vi "enableRtAxis.vi"(8 "error":errorcluster, 9 "enabled":bool=TRUE, 10 "axis":i32, 11 "connection ID":refnum<k5>) -> (0 "error out":errorcluster, 2 "axis_out":i32, 3 "connection ID out":refnum<k5>)   [LabVIEW 2016, in "sen_api.lvlib"]
doc: "Sets the real-time output of the specific measurement axis."
uses:
  sen_api.lvlib
panel:
  out "jsonRespIn":string
  out "JSON-response":string="{\"jsonrpc\":\"2.0\",\"method\":\"\",\"params\":[5,1.245,true,\"name\"],\"id\":\"1\"}"
  out "JSON request":string
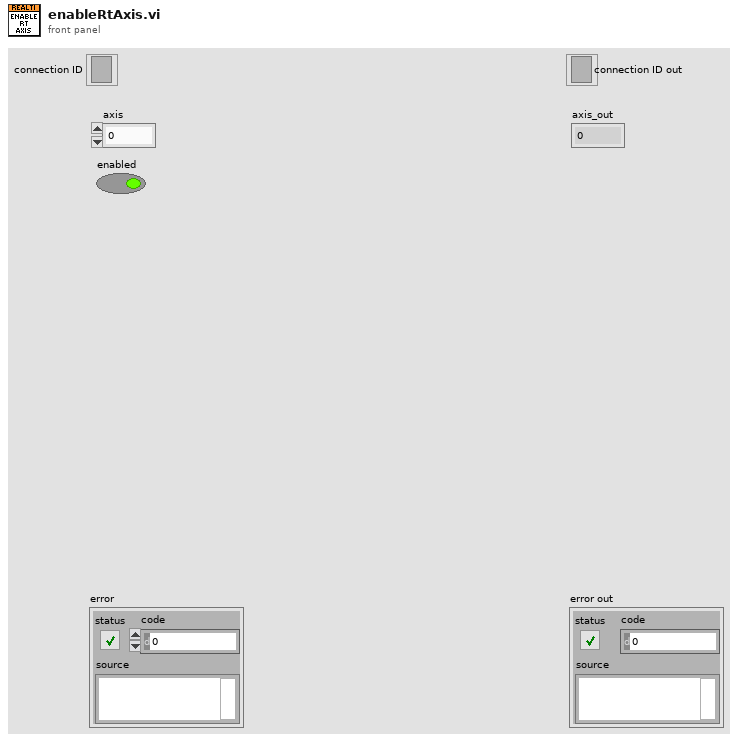
[diagram p1: front panel]
types:
  T1 = cluster{"jsonrpc":string, "method":string, "params":string[], "id":string, "api":i32, "pid":string}
  T2 = enum16{"Standard", "Buffered", "CRLF", "Immediate"}
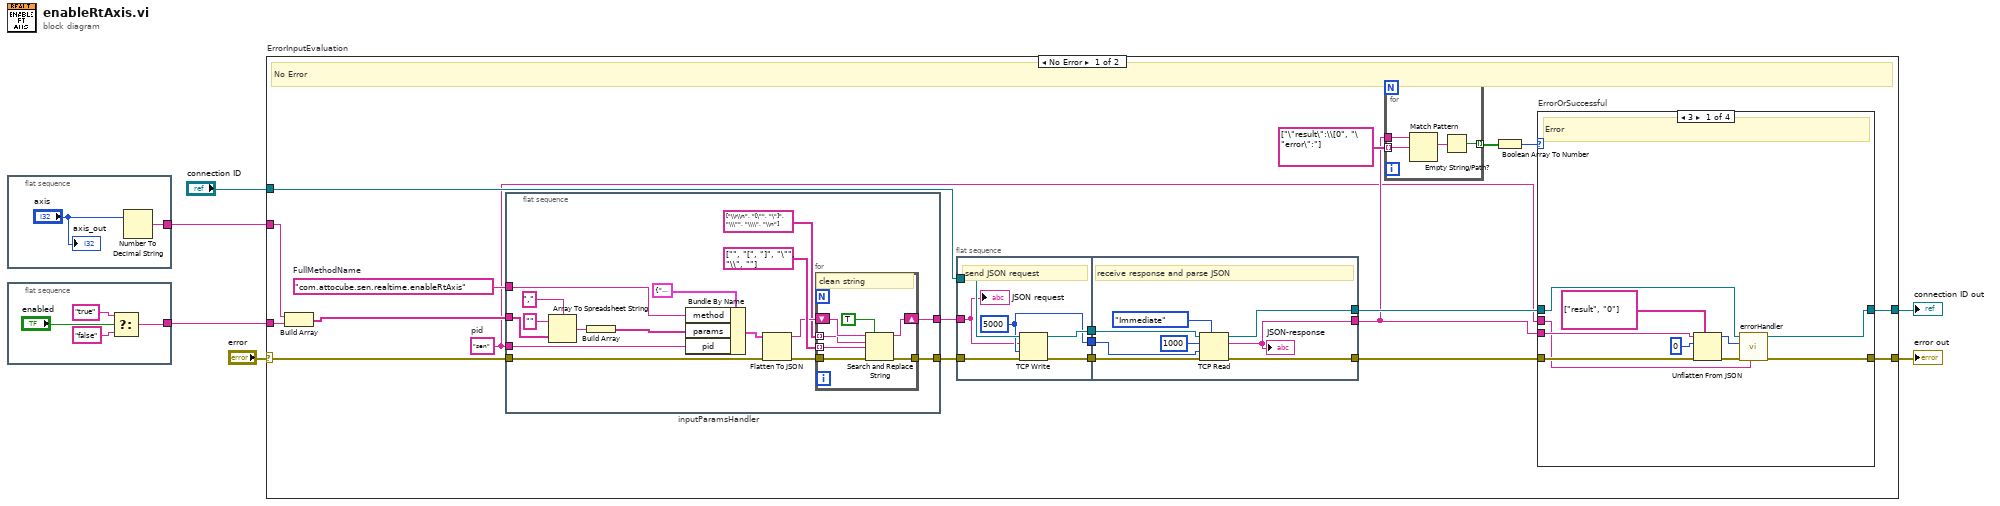
[diagram p0: block diagram]
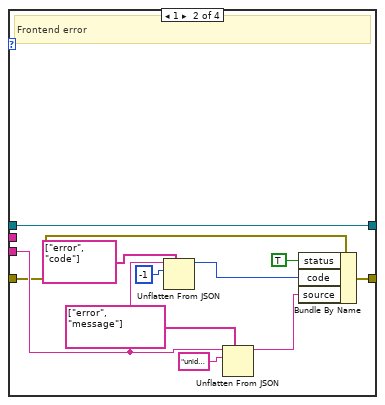
[diagram p2: hidden frame]
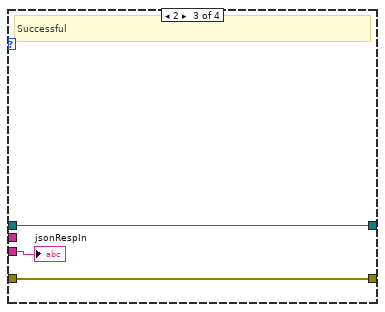
[diagram p3: hidden frame]
diagram:
  n1 = flat-sequence "in_axis" {
    tunnel: [w8] -> w2
    frame #0 {
      n2 = Number To Decimal String(number="axis") -> (decimal integer string=w8:string)  [unwired: 1 in]
      "axis_out" <- "axis"
    }
  }
  n3 = flat-sequence "in_bool" {
    tunnel: [w9] -> w1
    frame #0 {
      n4 = Select(t="true" ("Base"), s="enabled", f="false" ("Base")) -> (s? t:f=w9:string)
    }
  }
  n5 = case "ErrorInputEvaluation" shown="No Error" "error" {
    selector: "error" -> [w19 w100]
    tunnel: "connection ID" -> [w29 w101]
    tunnel: [w21 w100] -> w5
    tunnel: [w22 w101] -> w4
    tunnel: w2 -> [w14 _]
    tunnel: w1 -> [w13 _]
    frame No Error {
      w15 = "sen"  # pid
      w20 = "com.attocube.sen.realtime.enableRtAxis"  # FullMethodName
      # "No Error"
      n6 = Build Array ("ParametersArrayString")(w14, w13) -> (w18:string[])
      n7 = flat-sequence "inputParamsHandler" {
        tunnel: [w36] -> w17
        tunnel: w18 -> [w43]
        tunnel: w19 -> [w41]
        tunnel: [w38] -> w16
        tunnel: w20 -> [w44]
        tunnel: w15 -> [w33]
        frame #0 {
          n8 = Array To Spreadsheet String(delimiter (Tab)=",", array=w43, 3:"" ("format string")) -> (spreadsheet string=w46:string)
          n9 = Build Array "Build Array"(w46) -> (w42:string[])
          n10 = Bundle By Name(cluster=T1 {"jsonrpc"="2.0", "method"="com.attocube.amc.res.setRESReadOutFreq", "params"=[], "id"="1", "api"=2, "pid"=""}, "method"=w44, "params"=w42, "pid"=w33) -> (w45:T1)
          n11 = Flatten To JSON(anything=w45, error in (no error)=w41) -> (JSON string=w37:string, 11:w39:errorcluster)  [unwired: 1 in]
          n12 = for {
            tunnel: string[] ["\\r\\n", "[\"", "\"]", "\\\"", "\\\\", "\\n"] ("search string") -> [w52] mode=indexing
            tunnel: string[] ["", "[", "]", "\"", "\\", ""] ("replace string (\"\")") -> [w51] mode=indexing
            shift-right: [w54] -> w36
            shift-left: w37 -> [w53]
            tunnel: w39 -> [w50]
            tunnel: [w49] -> w38
            # "clean string"
            n13 = Search and Replace String(replace all?=TRUE ("replace all? (F)"), input string=w53, search string=w52, replace string=w51, error in=w50) -> (result string=w54:string, error out=w49:errorcluster)  [unwired: 3 in, 2 out]
          }
        }
      }
      n14 = flat-sequence {
        tunnel: w29 -> [w91]
        tunnel: [w89] -> w32
        tunnel: [w90] -> w31
        tunnel: w16 -> [w86]
        tunnel: [w88] -> w30
        tunnel: w17 -> [w87]
        tunnel: [w95] -> w25
        tunnel: w32 -> [w97]
        tunnel: w31 -> [w96]
        tunnel: [w93] -> w24
        tunnel: w30 -> [w94]
        tunnel: [w92] -> w23
        frame #0 {
          w88 = 5000 ("timeout ms (25000)")
          # "send JSON request"
          n15 = TCP Write(connection ID=w91, data in=w87, error in (no error)=w86, 9:w88) -> (connection ID out=w89:refnum<k5>, error out=w90:errorcluster)  [unwired: 1 out]
          "JSON request" <- w87
        }
        frame #1 {
          # "receive response and parse JSON"
          n16 = TCP Read(connection ID=w97, bytes to read=1000, error in (no error)=w96, 7:T2."Immediate" ("mode (standard)"), 9:w94) -> (connection ID out=w95:refnum<k5>, data out=w92:string, error out=w93:errorcluster)
          "JSON-response" <- w92
        }
      }
      n17 = for {
        tunnel: string[] ["\"result\":\\[0", "\"error\":"] ("path") -> [w58] mode=indexing
        tunnel: [w56] -> w27 mode=indexing
        tunnel: w23 -> [w59]
        n18 = Match Pattern(string=w59, regular expression=w58) -> (match substring=w57:string)  [unwired: 1 in, 3 out]
        n19 = Empty String/Path?(string/path=w57) -> (empty?=w56:bool)
      }
      n20 = Boolean Array To Number(Boolean array=w27) -> (number=w26:u32)
      n21 = case "ErrorOrSuccessful" shown="3" w26 {
        tunnel: w23 -> [w63 w72 w81 _]
        tunnel: w25 -> [w67 w70 w83 w85]
        tunnel: [w65 w70 w83 w85] -> w22
        tunnel: [w66 w73 w82 w84] -> w21
        tunnel: w24 -> [w69 w71 w82 w84]
        tunnel: w15 -> [w60 _ _ _]
        frame 3 {
          # "Error"
          n22 = Unflatten From JSON(path=string[] ["result", "0"], JSON string=w63, type and defaults=0, error in (no error)=w69) -> (value=w61:i32, error out=w68:errorcluster)  [unwired: 3 in]
          n23 = call "errorHandler.vi"("pid"=w60, "error in"=w68, "errNbr"=w61, "connection ID"=w67) -> ("error out 2"=w66:errorcluster, "connection ID out"=w65:refnum<k5>)  [unwired: 6 in]
        }
        frame 1 {
          # "Frontend error"
          n24 = Unflatten From JSON(path=string[] ["error", "code"], JSON string=w72, type and defaults=-1) -> (value=w79:i32)  [unwired: 4 in, 1 out]
          n25 = Unflatten From JSON(path=string[] ["error", "message"], JSON string=w72, type and defaults="unidentified error") -> (value=w80:string)  [unwired: 4 in, 1 out]
          n26 = Bundle By Name(cluster=w71, "status"=TRUE, "code"=w79, "source"=w80) -> (w73:errorcluster)
        }
        frame 2 {
          # "Successful"
          "jsonRespIn" <- w81
        }
        frame Default {
          # "NoResponse"
        }
      }
    }
    frame Error {
      # "Error"
    }
  }
  "error out" <- w5
  "connection ID out" <- w4
